vi "SubVI_Flash Detection_Image Process #.vi"(5 "Method":T1(ring), 7 "Image Register Name":string="untitled", 8 "Error in":errorcluster, 9 "Divider":sgl format="%.2f", 10 "Kernel Size":i32=3 min=3 max=201 step=2, 11 "Image Src In":T2) -> (0 "Error out":errorcluster, 2 "Image Dst Out":T2, 3 "Image Src Out":T2)   [LabVIEW 2013]
uses:
  <vilib>/vision/Image Controls.llb/IMAQ Image.ctl
  <vilib>/vision/NI_Vision_Development_Module.lvlib
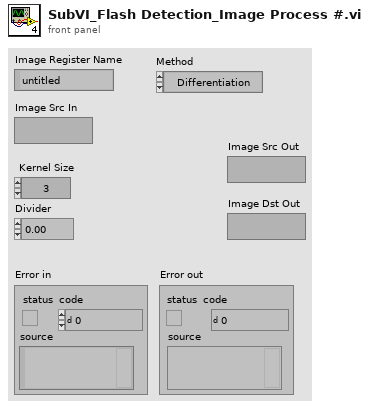
[diagram p1: front panel]
types:
  T1 = enum32{"Differentiation", "Gradient", "Prewitt", "Roberts", "Sigma", "Sobel"}
  T2 = typedef "IMAQ Image.ctl" = refnum<image>
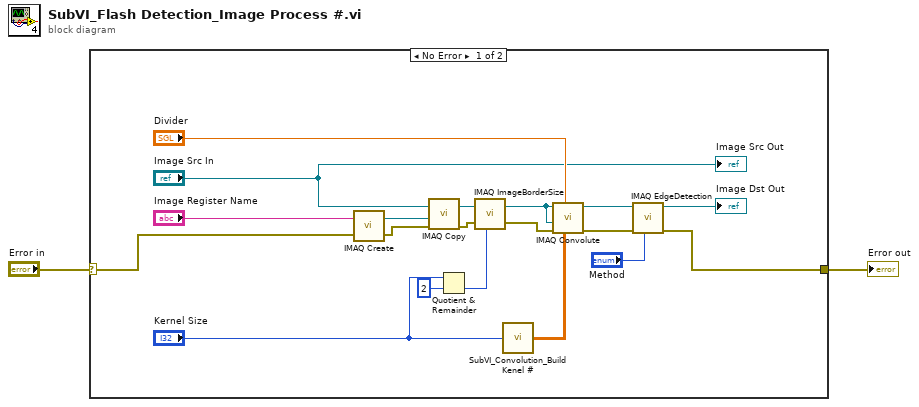
[diagram p0: block diagram]
diagram:
  n1 = case shown="No Error" "Error in" {
    selector: "Error in" -> [w11 w22]
    tunnel: [w4 w22] -> w1
    frame No Error {
      n2 = call "IMAQ Create"("Image Name"="Image Register Name", "error in (no error)"=w11) -> ("New Image"=w15:T2, "error out"=w10:errorcluster)  [unwired: 3 in]
      n3 = call "IMAQ Copy"("error in (no error)"=w10, "Image Dst"=w15, "Image Src"="Image Src In") -> ("error out"=w9:errorcluster, "Image Dst Out"=w14:T2)  [unwired: 3 in]
      n4 = Quotient & Remainder(x="Kernel Size", y=2) -> (floor(x/y)=w17:i32)  [unwired: 1 out]
      n5 = call "IMAQ ImageBorderSize"("Image"=w14, "Image border size in"=w17, "error in (no error)"=w9) -> ("Image Out"=w13:T2, "error out"=w8:errorcluster)  [unwired: 1 in, 1 out]
      n6 = call "SubVI_Convolution_Build Kenel #.vi"("Kernel Size"="Kernel Size") -> ("Kernel"=w21:sgl[][])
      n7 = call "IMAQ Convolute"("Kernel"=w21, "Divider (kernel sum)"="Divider", "error in (no error)"=w8, "Image Dst"=w13, "Image Src"=w13) -> ("error out"=w5:errorcluster, "Image Dst Out"=w7:T2)  [unwired: 5 in]
      n8 = call "IMAQ EdgeDetection"("Method"="Method", "error in (no error)"=w5, "Image Src"=w7) -> ("error out"=w4:errorcluster, "Image Dst Out"=→"Image Dst Out":T2)  [unwired: 3 in, 4 out]
      "Image Src Out" <- "Image Src In"
    }
    frame Error {
    }
  }
  "Error out" <- w1
